vi "ImageUriToObject.vi"(5 "image Path":path, 11 "error in (no error)":errorcluster) -> (6 ".Net Image":refnum<k24>, 15 "error out":errorcluster)   [LabVIEW 2018, in "DataGridView.lvclass"]
doc: "Converts a Image Uri to an .Net <b>System.Drawing.Image Object</b>"
uses:
  DataGridView.lvclass
  System.Drawing
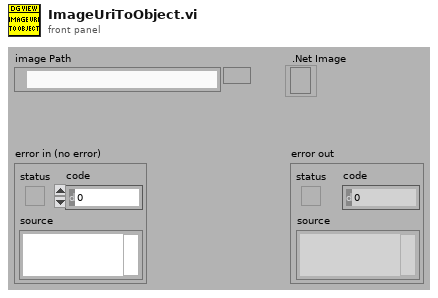
[diagram p1: front panel]
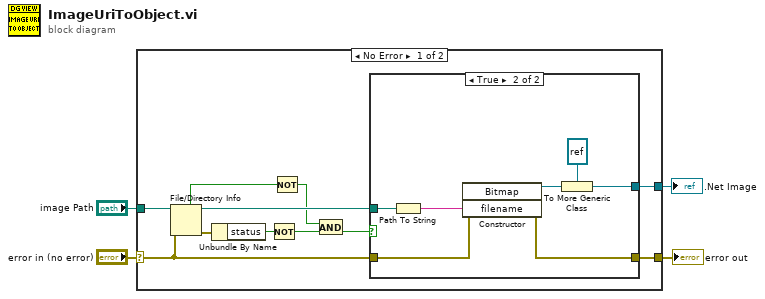
[diagram p0: block diagram]
diagram:
  n1 = case shown="No Error" "error in (no error)" {
    selector: "error in (no error)" -> [w10 w24]
    tunnel: [w11 w24] -> w3
    tunnel: "image Path" -> [w13 _]
    tunnel: [w5 _] -> w1
    frame No Error {
      n2 = File/Directory Info(path=w13, error in=w10) -> (path out=w9:path, directory=w7:bool, error out=w14:errorcluster)  [unwired: 4 out]
      n3 = Unbundle By Name(w14) -> ("status"=w15:bool)
      n4 = Not(x=w15) -> (.not. x?=w12:bool)
      n5 = Not(x=w7) -> (.not. x?=w6:bool)
      n6 = And(x=w6, y=w12) -> (x .and. y?=w8:bool)
      n7 = case shown="True" w8 {
        tunnel: w10 -> [w16 w21]
        tunnel: [w16 w20] -> w11
        tunnel: w9 -> [_ w23]
        tunnel: [_ w17] -> w5
        frame False {
        }
        frame True {
          n8 = Path To String(path=w23) -> (string=w22:string)
          n9 = constructor class="Bitmap"(error in=w21, "filename"=w22) -> (reference out=w18:refnum<k24>, error out=w20:errorcluster)  [unwired: 2 in, 2 out]
          n10 = To More Generic Class(target class=refnum<k24> refnum (".NET object"), reference=w18) -> (generic class reference=w17:refnum<k24>)
        }
      }
    }
    frame Error {
    }
  }
  "error out" <- w3
  ".Net Image" <- w1
